vi "Write Outgoing Bytes.vi"(8 "error in (no error)":errorcluster, 10 "Bytes":u8[](array[numeric]) format="%08b", 11 "WSConnection in":refnum<class "WebsocketsConnection.lvclass">) -> (0 "error out":errorcluster, 3 "WSConnection":refnum<class "WebsocketsConnection.lvclass">)   [LabVIEW 2013, in "MQTT_Websockets.lvlib" / "WebsocketsConnection.lvclass"]
uses:
  WebsocketsConnection.lvclass
  MQTT_Connection/Connection/Connection.lvclass/Connection.ctl
  WebsocketsConnection.lvclass/WebsocketsConnection.ctl
  <vilib>/MediaMongrels Ltd/WebSockets/WebSockets/WebSocket/WebSocket.lvclass
  MQTT_Connection/Connection/Connection.lvclass
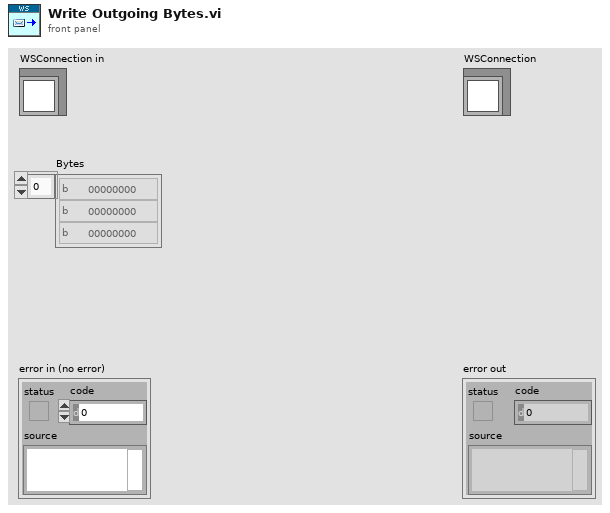
[diagram p1: front panel]
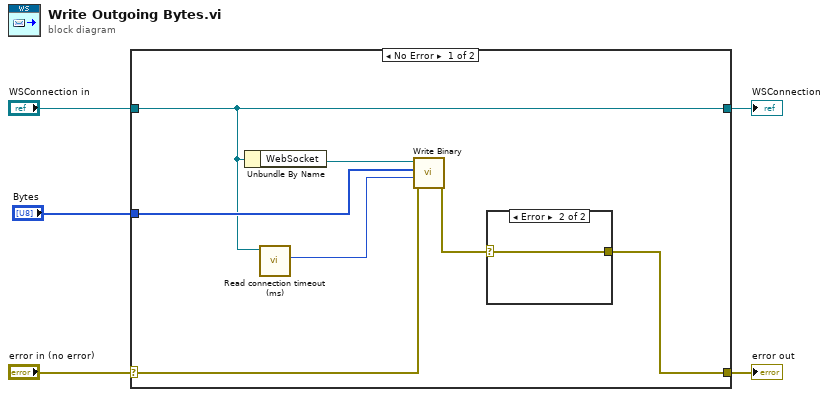
[diagram p0: block diagram]
diagram:
  n1 = case shown="No Error" "error in (no error)" {
    selector: "error in (no error)" -> [w9 w16]
    tunnel: [w12 w16] -> w4
    tunnel: [w7 w15] -> w2
    tunnel: "WSConnection in" -> [w7 w15]
    tunnel: "Bytes" -> [w10 _]
    frame No Error {
      n2 = Unbundle By Name(w7) -> ("WebSocket"=w11:refnum<class "WebSocket.lvclass">)
      n3 = call "Read connection timeout (ms).vi"("Connection in"=w7) -> ("connection timeout (ms)"=w6:i32)  [unwired: 8 in, 2 out]
      n4 = call-dynamic "Write Binary.vi"("error in (no error)"=w9, "timeout ms (5000)"=w6, "Binary Data"=w10, "WebSocket in"=w11) -> ("error out"=w8:errorcluster)  [unwired: 6 in, 1 out]
      n5 = case shown="Error" w8 {
        selector: w8 -> [w13 w14]
        tunnel: [w13 w14] -> w12
        frame No Error {
        }
        frame Error {
        }
      }
    }
    frame Error {
    }
  }
  "error out" <- w4
  "WSConnection" <- w2
